vi "Create Data Folders.vi"(10 "Experiment Indicator":string, 11 "username":string) -> (1 "Ageing box root path":path, 3 "Data Output Folder":path)   [LabVIEW 2011]
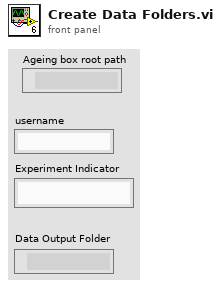
[diagram p1: front panel]
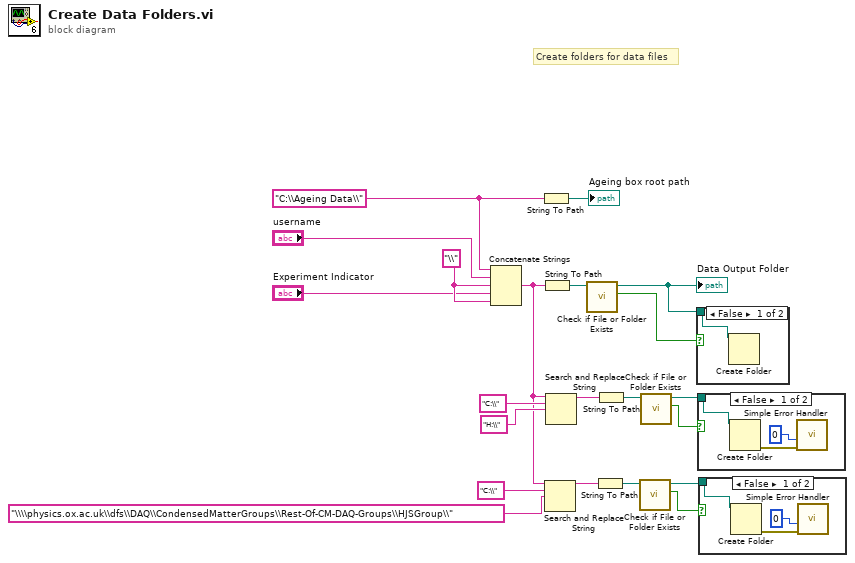
[diagram p0: block diagram]
diagram:
  w12 = "\\"
  w2 = "C:\\Ageing Data\\"
  # "Create folders for data files"
  n1 = Concatenate Strings(w2, "username", w12, "Experiment Indicator", w12) -> (w9:string)
  n2 = String To Path(string=w2) -> (path=→"Ageing box root path":path)
  n3 = String To Path(string=w9) -> (path=w20:path)
  n4 = Search and Replace String(input string=w9, search string="C:\\", replace string="\\\\physics.ox.ac.uk\\dfs\\DAQ\\CondensedMatterGroups\\Rest-Of-CM-DAQ-Groups\\HJSGroup\\") -> (result string=w13:string)  [unwired: 5 in, 3 out]
  n5 = Search and Replace String(input string=w9, search string="C:\\", replace string="H:\\") -> (result string=w17:string)  [unwired: 5 in, 3 out]
  n6 = call <vilib>:"Check if File or Folder Exists.vi"("path"=w20) -> ("file or folder exists?"=w21:bool, "dup path"=w4:path)  [unwired: 8 in, 1 out]
  "Data Output Folder" <- w4
  n7 = String To Path(string=w13) -> (path=w18:path)
  n8 = String To Path(string=w17) -> (path=w19:path)
  n9 = call <vilib>:"Check if File or Folder Exists.vi"("path"=w18) -> ("file or folder exists?"=w5:bool, "dup path"=w6:path)  [unwired: 8 in, 1 out]
  n10 = call <vilib>:"Check if File or Folder Exists.vi"("path"=w19) -> ("file or folder exists?"=w7:bool, "dup path"=w8:path)  [unwired: 8 in, 1 out]
  n11 = case shown="False" w21 {
    tunnel: w4 -> [w22 _]
    frame False {
      n12 = Create Folder(path (use dialog)=w22) -> ()  [unwired: 2 in, 3 out]
    }
    frame True {
    }
  }
  n13 = case shown="False" w7 {
    tunnel: w8 -> [w25 _]
    frame False {
      n14 = Create Folder(path (use dialog)=w25) -> (error out=w24:errorcluster)  [unwired: 2 in, 2 out]
      n15 = call <vilib>:"Simple Error Handler.vi"("type of dialog (OK msg:1)"=0, "error in (no error)"=w24) -> ()  [unwired: 3 in, 5 out]
    }
    frame True {
    }
  }
  n16 = case shown="False" w5 {
    tunnel: w6 -> [w28 _]
    frame False {
      n17 = Create Folder(path (use dialog)=w28) -> (error out=w27:errorcluster)  [unwired: 2 in, 2 out]
      n18 = call <vilib>:"Simple Error Handler.vi"("type of dialog (OK msg:1)"=0, "error in (no error)"=w27) -> ()  [unwired: 3 in, 5 out]
    }
    frame True {
    }
  }
